vi "Ramp_ITC.vi"(0 "RampTState":T1, 1 "Just read T":bool, 2 "Setpoint (K)":dbl format="%#_13g", 3 "Rate (K/min)":dbl format="%#_13g", 4 "ITC Info":T2={"ControlTITC"=0, "ControlTCh"=1, "SampleTITC"=0, "SampleTCh"=2}) -> ()   [LabVIEW 2016]
uses:
  Equipment/Oxford Software/Oxsoft/RAMP.LLB/RampTState.ctl
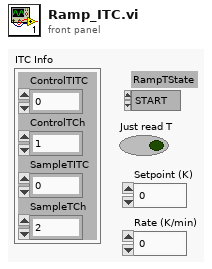
[diagram p1: front panel]
types:
  T1 = typedef "RampTState.ctl" = enum16{"START", "RUN"}
  T2 = cluster{"ControlTITC":i8, "ControlTCh":i8, "SampleTITC":i8, "SampleTCh":i8}
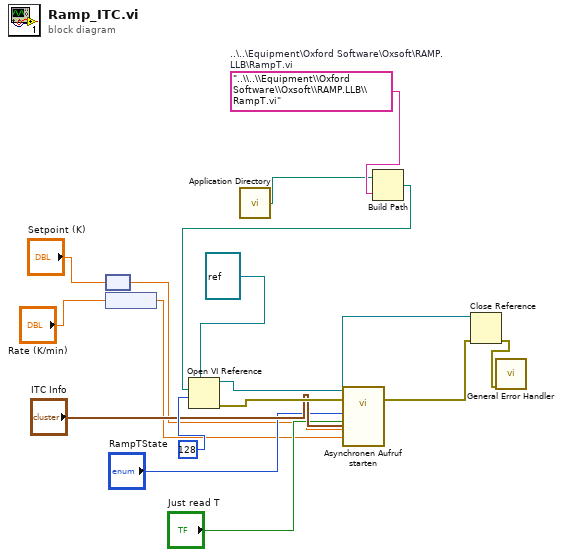
[diagram p0: block diagram]
diagram:
  w3 = "..\\..\\Equipment\\Oxford Software\\Oxsoft\\RAMP.LLB\\RampT.vi"  # ..\..\Equipment\Oxford Software\Oxsoft\RAMP.LLB\RampT.vi
  n1 = node("Setpoint (K)") -> (w6:dbl[unit])
  n2 = node("Rate (K/min)") -> (w4:dbl[unit])
  n3 = call <vilib>:"Application Directory.vi"() -> ("Application Directory"=w2:path)
  n4 = Build Path(base path=w2, name or relative path=w3) -> (appended path=w1:path)
  n5 = Open VI Reference ("VI-Referenz öffnen")(type specifier VI Refnum (for type only)=refnum<vi> refnum ("vi reference"), vi path=w1, options=128) -> (vi reference=w17:refnum<vi>, error out=w16:errorcluster)  [unwired: 3 in]
  n6 = call-by-ref "Asynchronen Aufruf starten"(reference=w17, error in=w16, "ITC Info"="ITC Info", "Rate"=w4, "Final Temperature"=w6, "JustReadTemperature"="Just read T", "RampTState"="RampTState") -> (reference out=w15:refnum<vi>, error out=w14:errorcluster)  [unwired: 5 out]
  n7 = Close Reference(reference=w15, error in (no error)=w14) -> (error out=w13:errorcluster)
  n8 = call <vilib>:"General Error Handler.vi"("error in (no error)"=w13) -> ()  [unwired: 10 in, 5 out]
